vi "PIDINIT.vi"(11 "setpoint":dbl format="%.2f") -> ()   [LabVIEW 2013]
uses:
  <vilib>/addons/control/pid/pid.llb/PID (DBL).vi
  <vilib>/addons/control/pid/NI_PID_pid.lvlib
panel:
  in  "y 2":dbl=0.59
  in  "PID Gains for distance":T1={"proportional gain (Kc)"=1.0, "integral time (Ti, min)"=0.01, "derivative time (Td, min)"=0.0} {"derivative time (Td, min)" format="%.3f"; "integral time (Ti, min)" format="%.3f"; "proportional gain (Kc)" format="%.3f"}
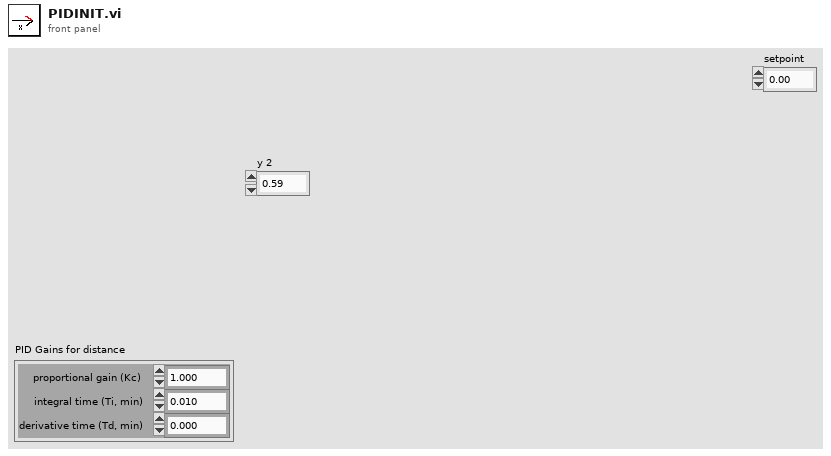
[diagram p1: front panel]
types:
  T1 = cluster{"proportional gain (Kc)":dbl, "integral time (Ti, min)":dbl, "derivative time (Td, min)":dbl}
  T2 = typedef "WPI_EncoderDevRef.ctl" = cluster{"DevStatus":errorcluster, "EncoderIndex":T3, "CounterIndex":T4, "DistancePerCount":dbl, "Decoding Type":T5}
  T3 = typedef "FPGA_EncoderIdx.ctl" = enum8{"Enc 0", "Enc 1", "Enc 2", "Enc 3", "Invalid"}
  T4 = typedef "FPGA_CounterCtrSystemIndex.ctl" = enum8{"Ctr 0", "Ctr 1", "Ctr 2", "Ctr 3", "Ctr 4", "Ctr 5", "Ctr 6", "Ctr 7", "Invalid"}
  T5 = typedef "WPI_EncoderType.ctl" = enum16{"1x", "2x", "4x"}
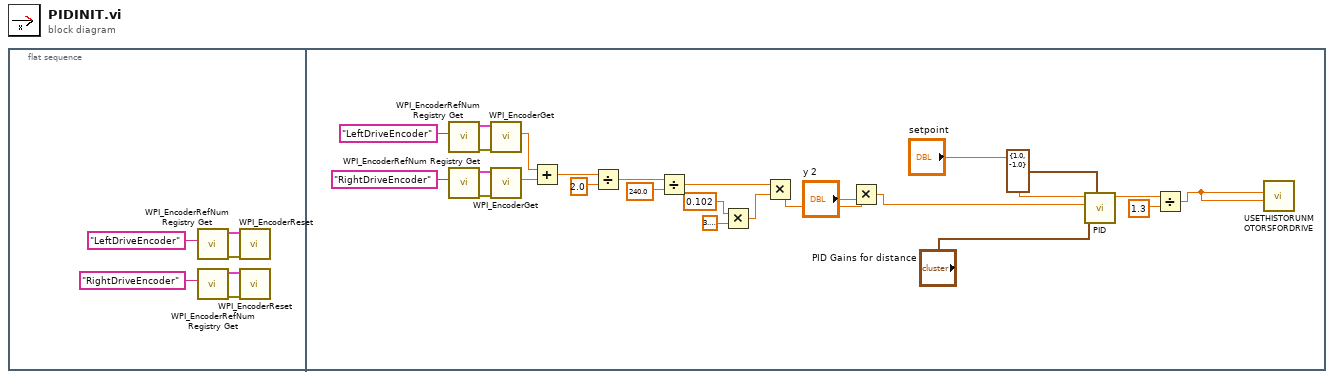
[diagram p0: block diagram]
diagram:
  n1 = flat-sequence {
    frame #0 {
      n2 = call <vilib>:"WPI_EncoderRefNum Registry Get.vi"("refnum name"="LeftDriveEncoder") -> ("error out"=w3:errorcluster, "EncoderDevRef"=w4:T2)  [unwired: 9 in]
      n3 = call <vilib>:"WPI_EncoderRefNum Registry Get.vi"("refnum name"="RightDriveEncoder") -> ("error out"=w5:errorcluster, "EncoderDevRef"=w6:T2)  [unwired: 9 in]
      n4 = call <vilib>:"WPI_EncoderReset.vi"("error in (no error)"=w3, "EncoderDevRef"=w4) -> ()  [unwired: 8 in, 2 out]
      n5 = call <vilib>:"WPI_EncoderReset.vi"("error in (no error)"=w5, "EncoderDevRef"=w6) -> ()  [unwired: 8 in, 2 out]
    }
    frame #1 {
      n6 = call <vilib>:"WPI_EncoderRefNum Registry Get.vi"("refnum name"="LeftDriveEncoder") -> ("error out"=w31:errorcluster, "EncoderDevRef"=w30:T2)  [unwired: 9 in]
      n7 = call <vilib>:"WPI_EncoderRefNum Registry Get.vi"("refnum name"="RightDriveEncoder") -> ("error out"=w29:errorcluster, "EncoderDevRef"=w28:T2)  [unwired: 9 in]
      n8 = call <vilib>:"WPI_EncoderGet.vi"("error in (no error)"=w31, "EncoderDevRef"=w30) -> ("Distance"=w25:dbl)  [unwired: 4 in, 5 out]
      n9 = call <vilib>:"WPI_EncoderGet.vi"("error in (no error)"=w29, "EncoderDevRef"=w28) -> ("Distance"=w14:dbl)  [unwired: 4 in, 5 out]
      n10 = Add(x=w25, y=w14) -> (x+y=w24:dbl)
      n11 = Divide(x=w24, y=2.0) -> (x/y=w20:dbl)
      n12 = Divide(x=w20, y=240.0) -> (x/y=w16:dbl)
      n13 = Multiply(x=0.102, y=3.141592653589793) -> (x*y=w18:dbl)
      n14 = Multiply(x=w16, y=w18) -> (x*y=w12:dbl)
      n15 = Multiply(x=w12, y="y 2") -> (x*y=w9:dbl)
      n16 = call-poly <vilib>:"PID.vi"("output range"=cluster{"output high":dbl, "output low":dbl} {"output high"=1.0, "output low"=-1.0}, "PID gains"="PID Gains for distance", "process variable"=w9, "setpoint"="setpoint") -> ("output"=w17:dbl)  [unwired: 6 in, 1 out]
      n17 = Divide(x=w17, y=1.3) -> (x/y=w8:dbl)
      n18 = call "USETHISTORUNMOTORSFORDRIVE.vi"("Y axis value"=w8, "X axis value"=w8) -> ()  [unwired: 10 in]
    }
  }
